vi "FunctionGeneratorMatrix_Calculate.vi"(9 "Input Value":dbl, 11 "FUNCTION_GENERATOR_MATRIX":T1) -> (3 "Output Matrix":T2)   [LabVIEW 2019, in "Trajectory_Library.lvlib"]
doc: "Calculate the output Y value for the provided X. This is done by interpolating through an array of X and Y pairs. The pairs must be ordered in increasing X value. (The Add function ensures that the X values are sorted properly.)\n\nInputs:\n - Function_Generator Matrix -- function generator data structure\n - Input Value -- The input value. \n\nOutputs:\n - Output Value -- Output matrix calcuated from the input value."
uses:
  Trajectory_Library.lvlib
  <vilib>/Analysis/Matrix/Datatypes/RealMatrix.ctl
  TypeDef/FUNCTION_GENERATOR_MATRIX.ctl
  <vilib>/Analysis/Matrix/Numeric/Subtract/Subtract - RM,RM.vi
  <vilib>/Analysis/Matrix/Numeric/Multiply/Multiply - RM,R.vi
  <vilib>/Analysis/Matrix/Numeric/Add/Add - RM,RM.vi
  <vilib>/gmath/NI_Gmath.lvlib
  <vilib>/Analysis/Matrix/NI_Matrix.lvlib
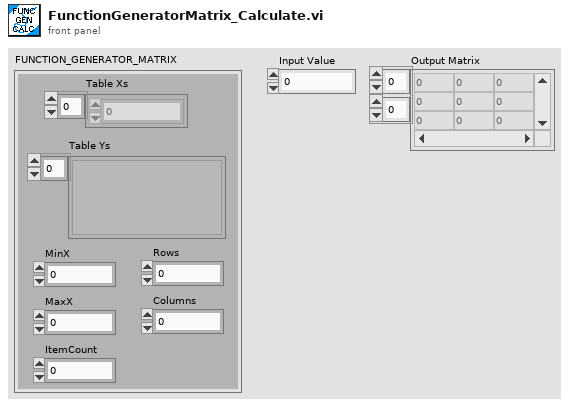
[diagram p1: front panel]
types:
  T1 = typedef "Trajectory_Library.lvlib/FUNCTION_GENERATOR_MATRIX.ctl" = cluster{"Table Xs":dbl[], "Table Ys":variant[], "MinX":dbl, "MaxX":dbl, "ItemCount":i32, "Rows":i32, "Columns":i32}
  T2 = typedef "NI_Matrix.lvlib/RealMatrix.ctl" = dbl[][]
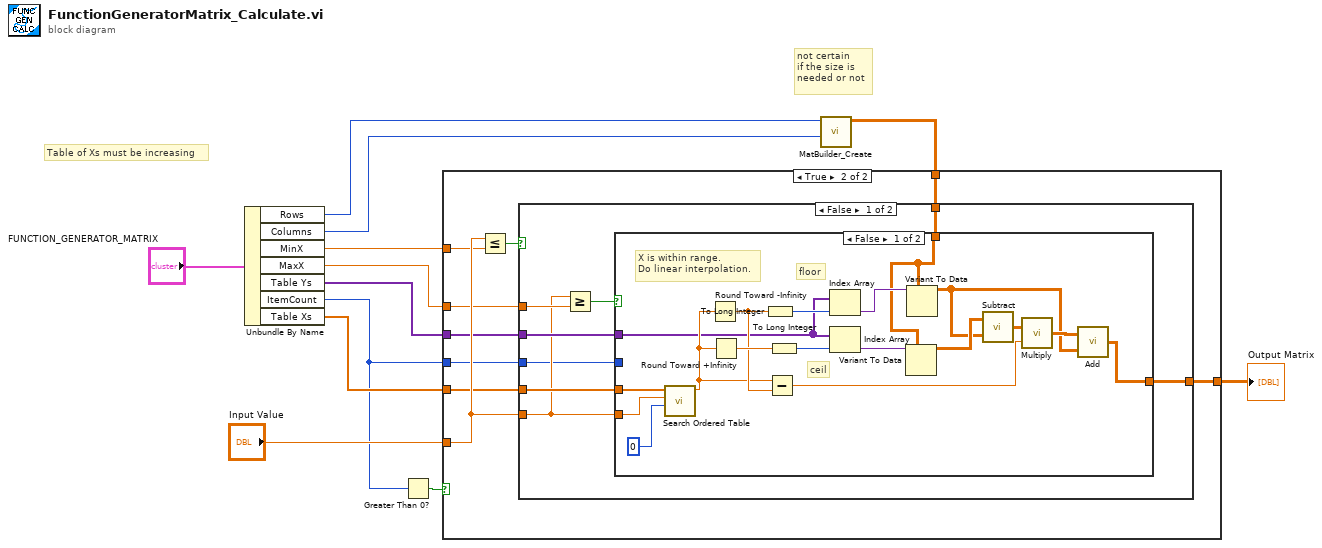
[diagram p0: block diagram]
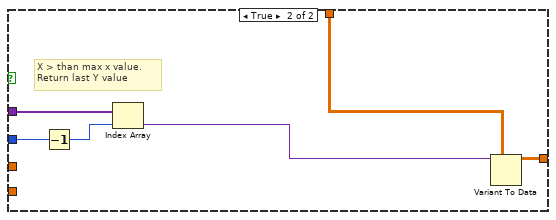
[diagram p3: hidden frame]
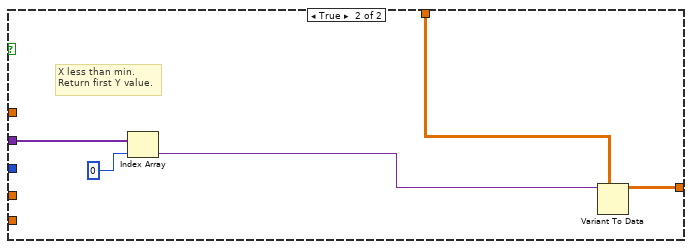
[diagram p4: hidden frame]
diagram:
  # "not certain\nif the size is\nneeded or not"
  # "Table of Xs must be increasing"
  n1 = Unbundle By Name("FUNCTION_GENERATOR_MATRIX") -> ("Rows"=w4:i32, "Columns"=w3:i32, "MinX"=w10:dbl, "MaxX"=w9:dbl, "Table Ys"=w7:variant[], "ItemCount"=w5:i32, "Table Xs"=w8:dbl[])
  n2 = Greater Than 0?(x=w5) -> (x > 0?=w6:bool)
  n3 = call "MatBuilder_Create.vi"("Columns"=w3, "Rows"=w4) -> ("output matrix"=w2:T2)  [unwired: 9 in]
  n4 = case shown="True" w6 {
    tunnel: "Input Value" -> [_ w21]
    tunnel: [w13 w20] -> w1
    tunnel: w10 -> [_ w19]
    tunnel: w9 -> [_ w18]
    tunnel: w5 -> [_ w17]
    tunnel: w8 -> [_ w16]
    tunnel: w7 -> [_ w15]
    tunnel: w2 -> [w13 w14]
    frame False {
    }
    frame True {
      n5 = Less Or Equal?(x=w21, y=w19) -> (x <= y?=w22:bool)
      n6 = case shown="False" w22 {
        tunnel: w15 -> [w28 w59]
        tunnel: [w24 w57] -> w20
        tunnel: w21 -> [w26 _]
        tunnel: w18 -> [w30 _]
        tunnel: w16 -> [w27 _]
        tunnel: w17 -> [w25 _]
        tunnel: w14 -> [w23 w55]
        frame False {
          n7 = Greater Or Equal?(x=w26, y=w30) -> (x >= y?=w29:bool)
          n8 = case shown="False" w29 {
            tunnel: w28 -> [w40 w54]
            tunnel: w27 -> [w47 _]
            tunnel: w26 -> [w46 _]
            tunnel: w25 -> [_ w53]
            tunnel: [w31 w51] -> w24
            tunnel: w23 -> [w37 w49]
            frame False {
              # "ceil"
              # "floor"
              # "X is within range.  \nDo linear interpolation."
              n9 = call <vilib>:"Search Ordered Table.vi"("starting index"=0, "x value"=w46, "ordered x array"=w47) -> ("fractional index"=w41:dbl)  [unwired: 8 in]
              n10 = Round Toward -Infinity(1:w41) -> (0:w42:dbl)
              n11 = Round Toward +Infinity(x=w41) -> (ceil(x): smallest int >= x=w43:dbl)
              n12 = To Long Integer(number=w42) -> (32bit integer=w45:i32)
              n13 = Subtract(x=w41, y=w42) -> (x-y=w34:dbl)
              n14 = To Long Integer(number=w43) -> (32bit integer=w44:i32)
              n15 = Index Array(array=w40, index=w45) -> (element=w38:variant)
              n16 = Index Array(array=w40, index=w44) -> (element=w39:variant)
              n17 = Variant To Data(type=w37, Variant=w39) -> (data=w36:T2)  [unwired: 1 in, 1 out]
              n18 = Variant To Data(type=w37, Variant=w38) -> (data=w32:T2)  [unwired: 1 in, 1 out]
              n19 = call-poly <vilib>:"Subtract.vi"("Real Matrix B"=w32, "Real Matrix A"=w36) -> ("A - B"=w35:T2)
              n20 = call-poly <vilib>:"Multiply.vi"("Real Scalar c"=w34, "Real Matrix A"=w35) -> ("A * c"=w33:T2)
              n21 = call-poly <vilib>:"Add.vi"("Real Matrix B"=w32, "Real Matrix A"=w33) -> ("A + B"=w31:T2)
            }
            frame True {
              # "X > than max x value.   \nReturn last Y value"
              n22 = Decrement(x=w53) -> (x-1=w52:i32)
              n23 = Index Array(array=w54, index=w52) -> (element=w50:variant)
              n24 = Variant To Data(type=w49, Variant=w50) -> (data=w51:T2)  [unwired: 1 in, 1 out]
            }
          }
        }
        frame True {
          # "X less than min.   \nReturn first Y value."
          n25 = Index Array(array=w59, index=0) -> (element=w56:variant)
          n26 = Variant To Data(type=w55, Variant=w56) -> (data=w57:T2)  [unwired: 1 in, 1 out]
        }
      }
    }
  }
  "Output Matrix" <- w1
